vi "Evaluator_init.vi"(0 "Evaluator in":refnum<class "Evaluator.lvclass">, 5 "ZoneDVR":refnum<data-value>, 7 "BallDVR":refnum<data-value>, 9 "FieldDVR":refnum<data-value>, 11 "error in (no error)":errorcluster) -> (4 "Evaluator out":refnum<class "Evaluator.lvclass">, 15 "error out":errorcluster)   [LabVIEW 2023, in "Evaluator.lvclass"]
uses:
  Evaluator.lvclass
  Zone_class/Zone.lvclass
  Field_class/Field.lvclass
  Ball_class/Ball.lvclass
  Objectives.ctl
  TestObjetive/TestObjetive.lvclass
  C:/Users/ebert/Documents/codes/SSL/repo/SSL_AI/Objective_class/Objective.lvclass
  Evaluator.lvclass/Evaluator.ctl
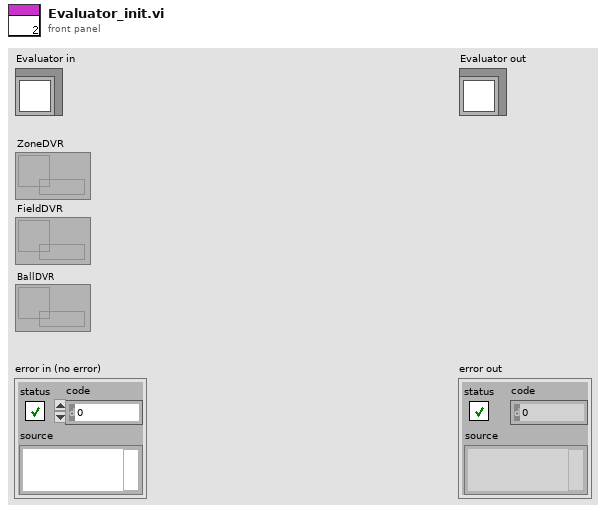
[diagram p1: front panel]
types:
  T1 = typedef "Evaluator.lvclass/Objectives.ctl" = enum16{"testObjective"}
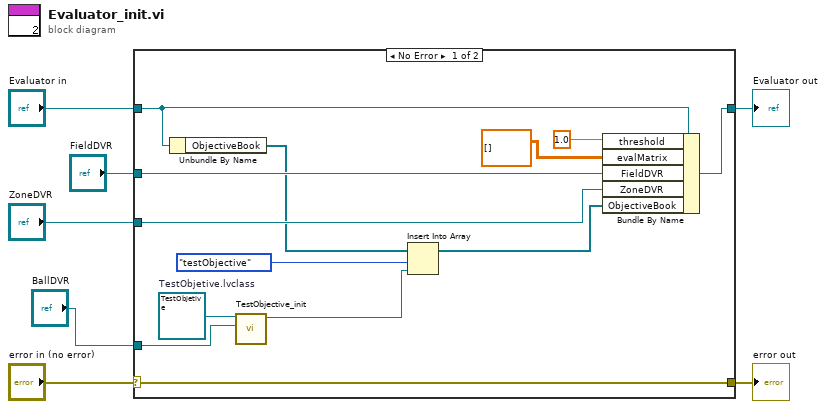
[diagram p0: block diagram]
diagram:
  n1 = case shown="No Error" "error in (no error)" {
    selector: "error in (no error)" -> [w20 w22]
    tunnel: [w20 w22] -> w6
    tunnel: [w19 w21] -> w4
    tunnel: "Evaluator in" -> [w13 w21]
    tunnel: "ZoneDVR" -> [w15 _]
    tunnel: "FieldDVR" -> [w17 _]
    tunnel: "BallDVR" -> [w8 _]
    frame No Error {
      w10 = refnum<class "TestObjetive.lvclass"> refnum  # TestObjetive.lvclass
      n2 = Unbundle By Name(w13) -> ("ObjectiveBook"=w12:refnum<class "Objective.lvclass">[])
      n3 = call-dynamic "TestObjective_init.vi"("BallDVR"=w8, "TestObjetive in"=w10) -> ("TestObjetive out"=w9:refnum<class "TestObjetive.lvclass">)  [unwired: 8 in, 1 out]
      n4 = Insert Into Array(array=w12, index=Objectives."testObjective" ("Objective"), new element=w9) -> (w11:refnum<class "Objective.lvclass">[])
      n5 = Bundle By Name(cluster=w13, "threshold"=1.0, "evalMatrix"=dbl[][] [], "FieldDVR"=w17, "ZoneDVR"=w15, "ObjectiveBook"=w11) -> (w19:refnum<class "Evaluator.lvclass">)
    }
    frame Error {
    }
  }
  "error out" <- w6
  "Evaluator out" <- w4
